vi "Make HTTP Request v4.vi"(5 "Request Options":T1={"request headers"=[], "request parameters"=[], "request body"="", "region handling"=enum."use region everywhere", "URL formatting"=enum."region."}, 7 "HTTP-Verb":string(combo)="GET", 8 "error in":errorcluster, 9 "URL Suffix":string, 10 "URL Prefix":string, 11 "AWS Core in":refnum<class "HTTP Request.lvclass">) -> (0 "error out":errorcluster, 1 "response body":string, 2 "response headers":string, 3 "AWS Core out":refnum<class "HTTP Request.lvclass">, 4 "Call Result":string)   [LabVIEW 2015, in "NI_AWS_Core.lvlib" / "HTTP Request.lvclass"]
uses:
  HTTP Request.lvclass
  Request Options.ctl
  Name Value Pair.ctl
  Region handling.ctl
  URL formatting.ctl
  HTTP Request.lvclass/HTTP Request.ctl
  Read Credentials.vi
  Read Service.vi
  Read Verify Server.vi
  <vilib>/httpClient/LabVIEWHTTPClient.lvlib
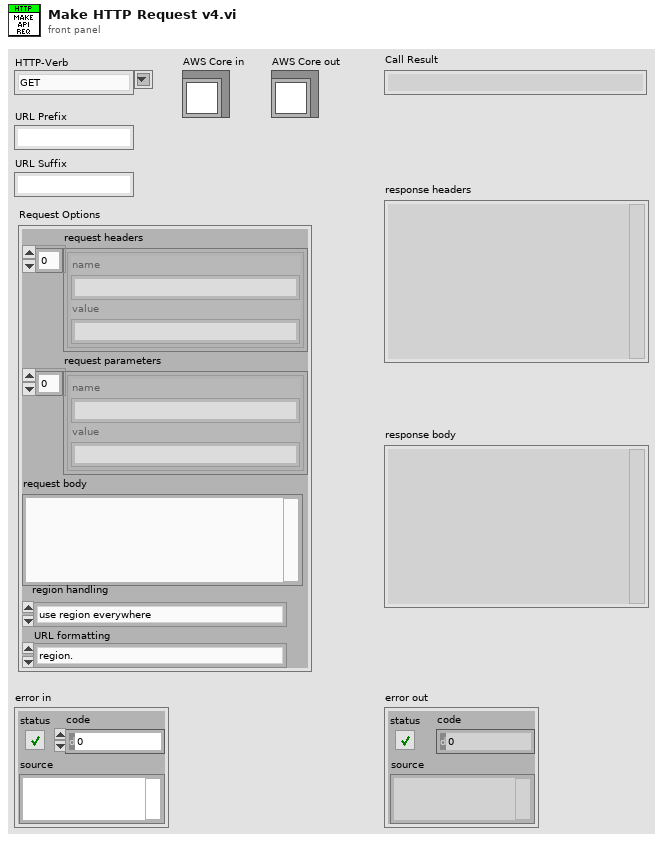
[diagram p1: front panel]
types:
  T1 = typedef "NI_AWS_Core.lvlib/HTTP Request.lvclass/Request Options.ctl" = cluster{"request headers":T2[], "request parameters":T2[], "request body":string, "region handling":T3, "URL formatting":T4}
  T2 = typedef "NI_AWS_Core.lvlib/HTTP Request.lvclass/Name Value Pair.ctl" = cluster{"name":string, "value":string}
  T3 = typedef "NI_AWS_Core.lvlib/HTTP Request.lvclass/Region handling.ctl" = enum16{"use region everywhere", "use region (authentication only)", "use region (URL only)", "ignore region everwhere"}
  T4 = typedef "NI_AWS_Core.lvlib/HTTP Request.lvclass/URL formatting.ctl" = enum16{"region-", "region."}
  T5 = typedef "AWS Core.lvlib/AWS Credentials.ctl" = cluster{"Access Key":string, "Secret Key":string}
  T6 = typedef "NI_AWS_Core.lvlib/HTTP Request.lvclass/Region.ctl" = enum16{"us-east-1", "us-east-2", "us-west-1", "us-west-2", "ap-northeast-1", "ap-northeast-2", "ap-southeast-1", "ap-southeast-2", "ca-central-1", "eu-central-1", "eu-west-1", "eu-west-2", "sa-east-1"}
  T7 = typedef "LabVIEWHTTPClient.lvlib/ClientHandle.ctl" = refnum<k1>
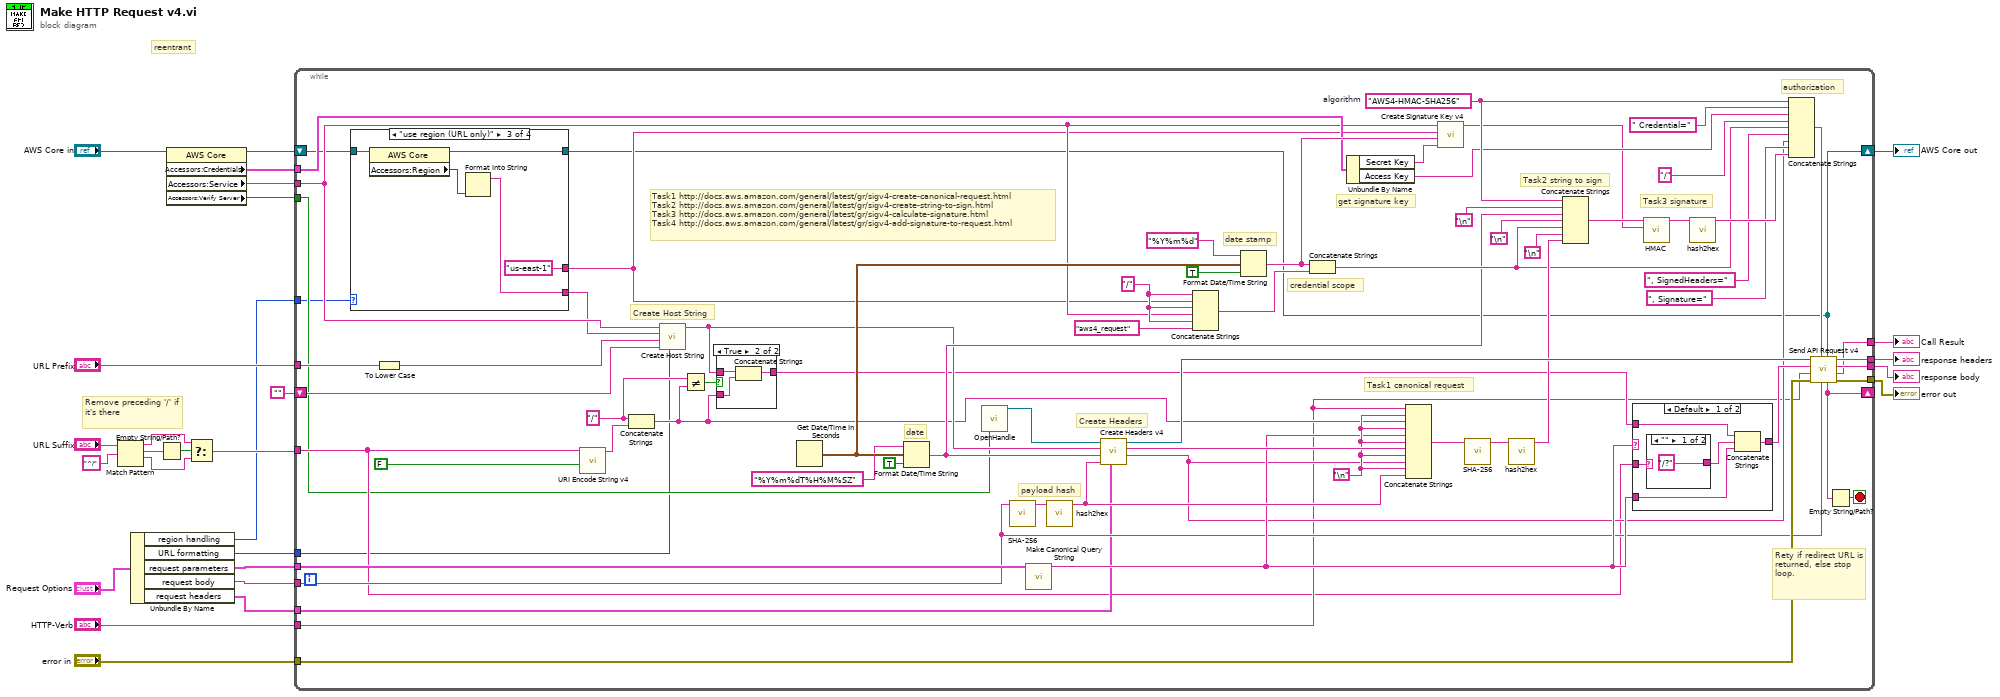
[diagram p0: block diagram]
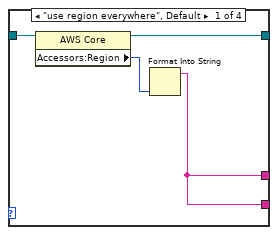
[diagram p2: hidden frame]
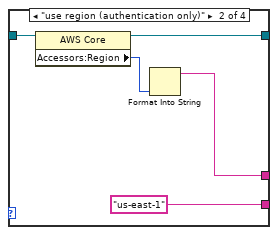
[diagram p3: hidden frame]
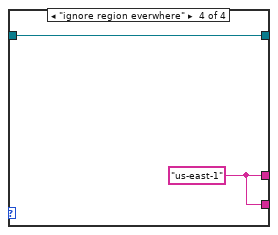
[diagram p4: hidden frame]
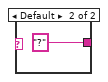
[diagram p6: hidden frame]
diagram:
  # "reentrant"
  # "Remove preceding '/' if it's there"
  n1 = Match Pattern(string="URL Suffix", regular expression="^/") -> (before substring=w21:string, match substring=w19:string, after substring=w22:string)  [unwired: 1 in, 1 out]
  n2 = Unbundle By Name("Request Options") -> ("region handling"=w3:T3, "URL formatting"=w2:T4, "request parameters"=w5:T2[], "request body"=w6:string, "request headers"=w4:T2[])
  n3 = Empty String/Path?(string/path=w19) -> (empty?=w20:bool)
  n4 = property class="AWS Core"(reference="AWS Core in") -> (reference out=w11:refnum<class "HTTP Request.lvclass">, "Accessors:Credentials"=w10:T5, "Accessors:Service"=w9:string, "Accessors:Verify Server"=w8:bool)  [unwired: 1 in, 1 out]
  n5 = Select(t=w21, s=w20, f=w22) -> (s? t:f=w17:string)
  n6 = while {
    tunnel: [w96] -> w27
    tunnel: [w49] -> w25
    tunnel: [w54] -> w24
    shift-right: [w53] -> _
    shift-left: "" ("Redirect endpoint") -> [w51]
    tunnel: [w50] -> w26
    tunnel: "error in" -> [w46]
    tunnel: w17 -> [w36]
    tunnel: "URL Prefix" -> [w42]
    tunnel: w5 -> [w41]
    tunnel: w6 -> [w40]
    tunnel: w4 -> [w39]
    tunnel: "HTTP-Verb" -> [w38]
    tunnel: w10 -> [w37]
    tunnel: w9 -> [w34]
    tunnel: w8 -> [w35]
    tunnel: w3 -> [w33]
    tunnel: w2 -> [w30]
    shift-right: [w28] -> w1
    shift-left: w11 -> [w29]
    stop <- w52 stop-if-true
    w59 = "/" ("string")
    w70 = "/" ("string")
    w88 = "AWS4-HMAC-SHA256"  # algorithm
    w66 = "\n"
    # "Rety if redirect URL is returned, else stop loop."
    # "Create Host String"
    # "Task1 canonical request"
    # "Create Headers"
    # "get signature key"
    # "Task1 http://docs.aws.amazon.com/general/latest/gr/sigv4-create-canonical-request.html\nTask2 http://docs.aws.amazon.com/general/latest/gr/sigv4-create-string-to-sign.html\nTask3 http://docs.aws.amazon.com/general/latest/gr/sigv4-calculate-signature.html\nTask4 http://docs.aws.amazon.com/general/latest/gr/sigv4-add-signature-to-request.html"
    # "date stamp"
    # "date"
    # "payload hash"
    # "authorization"
    # "Task3 signature"
    # "Task2 string to sign"
    # "credential scope"
    n7 = case shown="\"use region (URL only)\"" w33 {
      tunnel: [w97 w101 "us-east-1" ("x") w112] -> w32
      tunnel: [w97 "us-east-1" ("x") w106 w112] -> w31
      tunnel: w29 -> [w99 w103 w108 w111]
      tunnel: [w98 w102 w107 w111] -> w28
      frame "use region everywhere", Default {
        n8 = property class="AWS Core"(reference=w99) -> (reference out=w98:refnum<class "HTTP Request.lvclass">, "Accessors:Region"=w100:T6)  [unwired: 1 in, 1 out]
        n9 = Format Into String(w100) -> (resulting string=w97:string)  [unwired: 3 in, 1 out]
      }
      frame "use region (authentication only)" {
        n10 = property class="AWS Core"(reference=w103) -> (reference out=w102:refnum<class "HTTP Request.lvclass">, "Accessors:Region"=w104:T6)  [unwired: 1 in, 1 out]
        n11 = Format Into String(w104) -> (resulting string=w101:string)  [unwired: 3 in, 1 out]
      }
      frame "use region (URL only)" {
        n12 = property class="AWS Core"(reference=w108) -> (reference out=w107:refnum<class "HTTP Request.lvclass">, "Accessors:Region"=w109:T6)  [unwired: 1 in, 1 out]
        n13 = Format Into String(w109) -> (resulting string=w106:string)  [unwired: 3 in, 1 out]
      }
      frame "ignore region everwhere" {
        w112 = "us-east-1" ("x")
      }
    }
    n14 = To Lower Case(string=w42) -> (all lower case string=w47:string)
    n15 = call "URI Encode String v4.vi"("Encode /"=FALSE, "Un-encoded String"=w36) -> ("UriEncoded String"=w44:string)  [unwired: 9 in]
    n16 = Concatenate Strings(w59, w44) -> (w56:string)
    n17 = call "Create Host String.vi"("URL formatting"=w30, "Redirect Endpoint"=w51, "URL Prefix"=w47, "Region"=w31, "AWS Service"=w34) -> ("Host String"=w57:string)  [unwired: 6 in]
    n18 = Not Equal?(x=w59, y=w56) -> (x != y?=w58:bool)
    n19 = case shown="True" w58 {
      tunnel: w57 -> [w113 w116]
      tunnel: w56 -> [_ w115]
      tunnel: [w113 w114] -> w55
      frame False {
      }
      frame True {
        n20 = Concatenate Strings(w116, w115) -> (w114:string)
      }
    }
    n21 = Get Date/Time In Seconds() -> (seconds since 1Jan1904=w63:timestamp)
    n22 = Format Date/Time String(time format string (%c)="%Y%m%dT%H%M%SZ", seconds (now)=w63, UTC format=TRUE) -> (date/time string=w64:string)
    n23 = call <vilib>:"OpenHandle.vi"("verify server(true)"=w35) -> ("client handle out"=w67:T7)  [unwired: 13 in, 1 out]
    n24 = call "SHA-256.vi"("Message"=w40) -> ("Hash Value"=w80:string)  [unwired: 10 in]
    n25 = call "Make Canonical Query String.vi"("request parameters"=w41) -> ("canonical parameters"=w60:string)  [unwired: 10 in]
    n26 = call "hash2hex.vi"("hash string"=w80) -> ("hex string"=w65:string)  [unwired: 10 in]
    n27 = call "Create Headers v4.vi"("request headers"=w39, "RequestBody Payload"=w65, "date/time string"=w64, "Host"=w57, "Client Handle In"=w67) -> ("Signed Headers"=w48:string, "canonical headers"=w84:string, "Client Handle Out"=w94:T7)  [unwired: 3 in]
    n28 = Concatenate Strings(w70, w32, w70, w34, w70, "aws4_request" ("string")) -> (w71:string)
    n29 = Format Date/Time String(time format string (%c)="%Y%m%d", seconds (now)=w63, UTC format=TRUE) -> (date/time string=w77:string)
    n30 = Concatenate Strings(w77, w71) -> (w72:string)
    n31 = Unbundle By Name(w37) -> ("Secret Key"=w68:string, "Access Key"=w74:string)
    n32 = Concatenate Strings(w38, w66, w56, w66, w60, w66, w84, w66, w48, w66, w65) -> (w79:string)
    n33 = call "Create Signature Key v4.vi"("AWS Service"=w34, "Region"=w32, "date/time string"=w77, "Secret Key"=w68) -> ("Keyed-Hash"=w45:string)  [unwired: 6 in]
    n34 = call "SHA-256.vi"("Message"=w79) -> ("Hash Value"=w78:string)  [unwired: 10 in]
    n35 = call "hash2hex.vi"("hash string"=w78) -> ("hex string"=w87:string)  [unwired: 10 in]
    n36 = Concatenate Strings(w88, "\n", w64, "\n", w72, "\n", w87) -> (w76:string)
    n37 = case shown="Default" w60 {
      tunnel: [w121 w124] -> w61
      tunnel: w55 -> [w119 w124]
      tunnel: w60 -> [w120 _]
      tunnel: w36 -> [w117 _]
      frame Default {
        n38 = case shown="\"\"" w117 {
          tunnel: ["/?" ("string") "?" ("string")] -> w118
          frame "" {
          }
          frame Default {
          }
        }
        n39 = Concatenate Strings(w119, w118, w120) -> (w121:string)
      }
      frame "" {
      }
    }
    n40 = call "HMAC.vi"("Key"=w45, "Message"=w76) -> ("Keyed Hash"=w75:string)  [unwired: 9 in]
    n41 = call "hash2hex.vi"("hash string"=w75) -> ("hex string"=w93:string)  [unwired: 10 in]
    n42 = Concatenate Strings(w88, " Credential=", w74, "/", w72, ", SignedHeaders=", w48, ", Signature=", w93) -> (w95:string)
    n43 = call "Send API Request v4.vi"("AWS Core"=w28, "request body"=w40, "Authorization"=w95, "error in (no error)"=w46, "HTTP-Verb"=w38, "Host String"=w61, "Client Handle"=w94) -> ("error out"=w49:errorcluster, "Call Result"=w50:string, "response body"=w54:string, "response headers"=w96:string, "Redirect endpoint"=w53:string)
    n44 = Empty String/Path?(string/path=w53) -> (empty?=w52:bool)
  }
  "response headers" <- w27
  "response body" <- w24
  "error out" <- w25
  "Call Result" <- w26
  "AWS Core out" <- w1
